vi "String2StimParam.vi"(1 "string":string) -> (0 "stimulus parameters":T1)   [LabVIEW 2014]
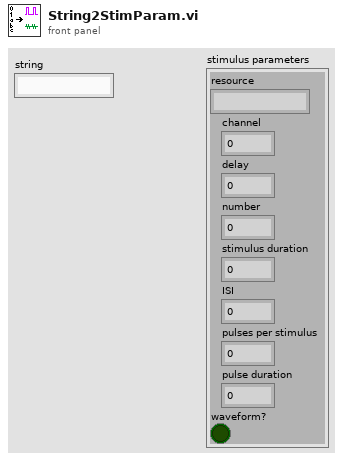
[diagram p1: front panel]
types:
  T1 = cluster{"resource":string, "channel":u16, "delay":dbl, "number":i32, "stimulus duration":dbl, "ISI":dbl, "pulses per stimulus":u16, "pulse duration":dbl, "waveform?":bool}
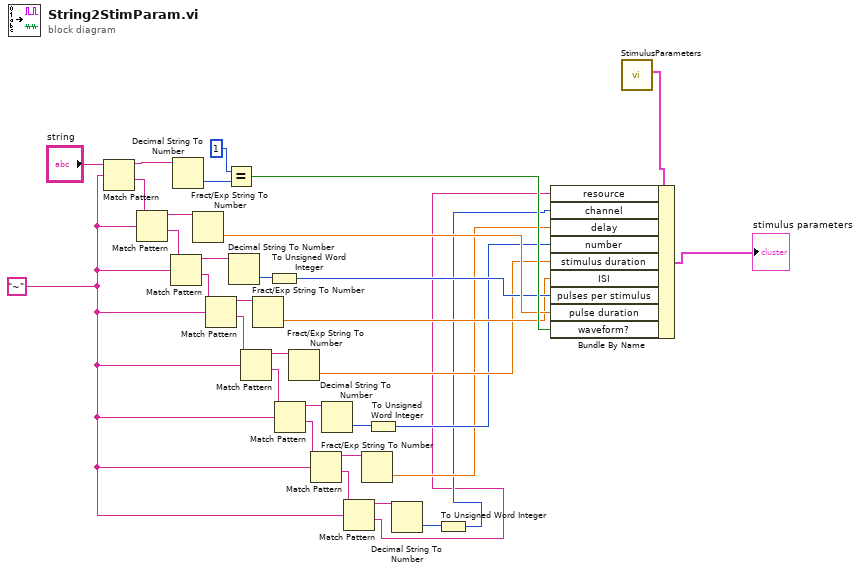
[diagram p0: block diagram]
diagram:
  w5 = "~"
  n1 = Match Pattern(string="string", regular expression=w5) -> (before substring=w30:string, after substring=w26:string)  [unwired: 1 in, 2 out]
  n2 = Match Pattern(string=w26, regular expression=w5) -> (before substring=w25:string, after substring=w23:string)  [unwired: 1 in, 2 out]
  n3 = Match Pattern(string=w23, regular expression=w5) -> (before substring=w22:string, after substring=w19:string)  [unwired: 1 in, 2 out]
  n4 = Decimal String To Number(string=w30) -> (number=w29:i32)  [unwired: 2 in, 1 out]
  n5 = Fract/Exp String To Number(string=w25) -> (number=w24:dbl)  [unwired: 3 in, 1 out]
  n6 = Match Pattern(string=w19, regular expression=w5) -> (before substring=w18:string, after substring=w16:string)  [unwired: 1 in, 2 out]
  n7 = Equal?(x=1, y=w29) -> (x = y?=w27:bool)
  n8 = Decimal String To Number(string=w22) -> (number=w21:i32)  [unwired: 2 in, 1 out]
  n9 = Match Pattern(string=w16, regular expression=w5) -> (before substring=w15:string, after substring=w13:string)  [unwired: 1 in, 2 out]
  n10 = Fract/Exp String To Number(string=w18) -> (number=w17:dbl)  [unwired: 3 in, 1 out]
  n11 = To Unsigned Word Integer(number=w21) -> (unsigned 16bit integer=w20:u16)
  n12 = Match Pattern(string=w13, regular expression=w5) -> (before substring=w12:string, after substring=w9:string)  [unwired: 1 in, 2 out]
  n13 = Fract/Exp String To Number(string=w15) -> (number=w14:dbl)  [unwired: 3 in, 1 out]
  n14 = Match Pattern(string=w9, regular expression=w5) -> (before substring=w8:string, after substring=w6:string)  [unwired: 1 in, 2 out]
  n15 = Decimal String To Number(string=w12) -> (number=w11:i32)  [unwired: 2 in, 1 out]
  n16 = Match Pattern(string=w6, regular expression=w5) -> (before substring=w4:string, after substring=w1:string)  [unwired: 1 in, 2 out]
  n17 = Fract/Exp String To Number(string=w8) -> (number=w7:dbl)  [unwired: 3 in, 1 out]
  n18 = To Unsigned Word Integer(number=w11) -> (unsigned 16bit integer=w10:u16)
  n19 = Decimal String To Number(string=w4) -> (number=w3:i32)  [unwired: 2 in, 1 out]
  n20 = To Unsigned Word Integer(number=w3) -> (unsigned 16bit integer=w2:u16)
  n21 = call "StimulusParameters.vi"() -> ("stimulus parameters"=w33:T1)  [unwired: 11 in]
  n22 = Bundle By Name(cluster=w33, "resource"=w1, "channel"=w2, "delay"=w7, "number"=w10, "stimulus duration"=w14, "ISI"=w17, "pulses per stimulus"=w20, "pulse duration"=w24, "waveform?"=w27) -> (→"stimulus parameters":T1)
